vi "1.vi"() -> ()   [LabVIEW 2015]
panel:
  out "Numérique 2":i32
  in  "Numérique":i32
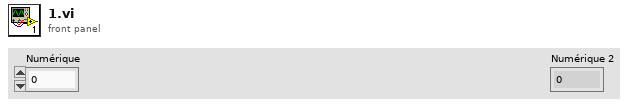
[diagram p1: front panel]
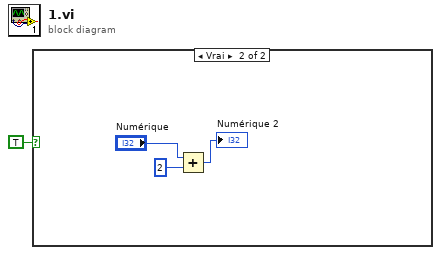
[diagram p0: block diagram]
diagram:
  n1 = case shown="Vrai" TRUE {
    frame False {
    }
    frame True {
      n2 = Add(x="Numérique", y=2) -> (x+y=→"Numérique 2":i32)
    }
  }
